vi "SR SIM921 Set Active Curve.vi"(4 "Error In":errorcluster, 5 "Curve #":i32, 6 "SIM Slot #":T1(radio), 7 "VISA session":refnum<visa-resource-name>) -> (0 "Error Out":errorcluster, 3 "dup VISA session":refnum<visa-resource-name>)   [LabVIEW 2025]
doc: "This VI reads a curve header from the LakeShore Model 370 AC Resistance Bridge and returns the parsed data.\nScott Hannahs, <sth@magnet.fsu.edu> NHMFL-FSU, May 2003\nAuthor: Scott Hannahs <sth@magnet.fsu.edu>\n\nThis software is licensed for use under the “MIT License\"\nCopyright (c) 2025 Scott Hannahs, sth@sth@magnet.sthnet.net\n\nPermission is hereby granted, free of charge, to any person obtaining a copy of this software and associated documentation files (the \"Software\"), to deal in the Software without restriction, including without limitation the rights to use, copy, modify, merge, publish, distribute, sublicense, and/or sell copies of the Software, and to permit persons to whom the Software is furnished to do so, subject to the following conditions: The above copyright notice and this permission notice shall be included in all copies or substantial portions of the Software.\n\nTHE SOFTWARE IS PROVIDED \"AS IS\", WITHOUT WARRANTY OF ANY KIND, EXPRESS OR IMPLIED, INCLUDING BUT NOT LIMITED TO THE WARRANTIES OF MERCHANTABILITY, FITNESS FOR A PARTICULAR PURPOSE AND NONINFRINGEMENT. IN NO EVENT SHALL THE AUTHORS OR COPYRIGHT HOLDERS BE LIABLE FOR ANY CLAIM, DAMAGES OR OTHER LIABILITY, WHETHER IN AN ACTION OF CONTRACT, TORT OR OTHERWISE, ARISING FROM, OUT OF OR IN CONNECTION WITH THE SOFTWARE OR THE USE OR OTHER DEALINGS IN THE SOFTWARE."
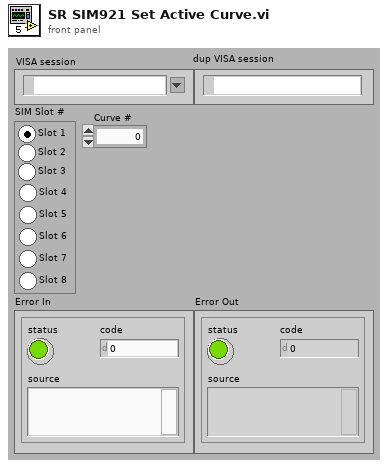
[diagram p1: front panel]
types:
  T1 = enum32{"Slot 1", "Slot 2", "Slot 3", "Slot 4", "Slot 5", "Slot 6", "Slot 7", "Slot 8"}
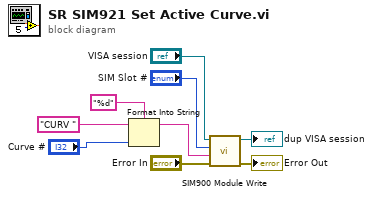
[diagram p0: block diagram]
diagram:
  n1 = Format Into String(format string="%d", initial string="CURV " ("String to Write"), "Curve #") -> (resulting string=w2:string)  [unwired: 1 in, 1 out]
  n2 = call "SIM900 Module Write.vi"("Error In"="Error In", "Query"=w2, "Slot"="SIM Slot #", "VISA Resource Name"="VISA session") -> ("Error Out"=→"Error Out":errorcluster, "dup VISA Session"=→"dup VISA session":refnum<visa-resource-name>)  [unwired: 6 in]
